vi "AMI_Measure_cDAQ.vi"(6 "error in (no error)":errorcluster, 7 "Index":i8) -> (0 "error out":errorcluster, 2 "resulting string 1":string="Set Temperatura 4.2K at 20K/min, FastSettle, Sweep&meas", 3 "Cancelled?":bool)   [LabVIEW 2017]
doc: "Use this template to create a dialog box. This template polls the state of the buttons on the front panel and does not use events. Use the Dialog Using Events template (not available in Base package) to create a dialog box with event handling."
panel:
  in  "Meas Time (s)":dbl=10.0
  in  "Measure Rate (s)":dbl=1.0 format="%.2f"
  in  "Averages":u16=10
  out "Channel 1":bool=TRUE
  out "Channel 2":bool=TRUE
  out "Channel 3":bool=TRUE
  out "Channel 4":bool=TRUE
  in  "Cancel":bool
  in  "OK":bool
  # "MEASURE cDAQ"
  # "Enero 2023 V2.1  a-sslcdms"
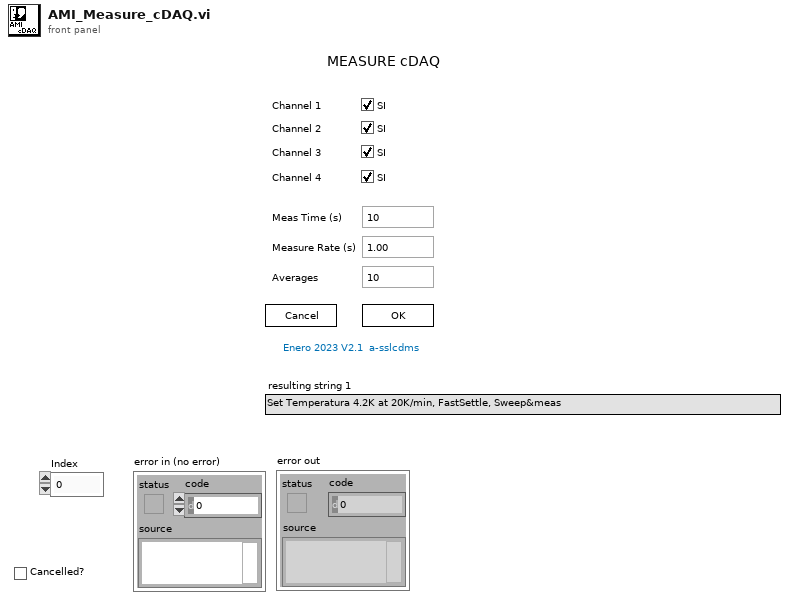
[diagram p1: front panel]
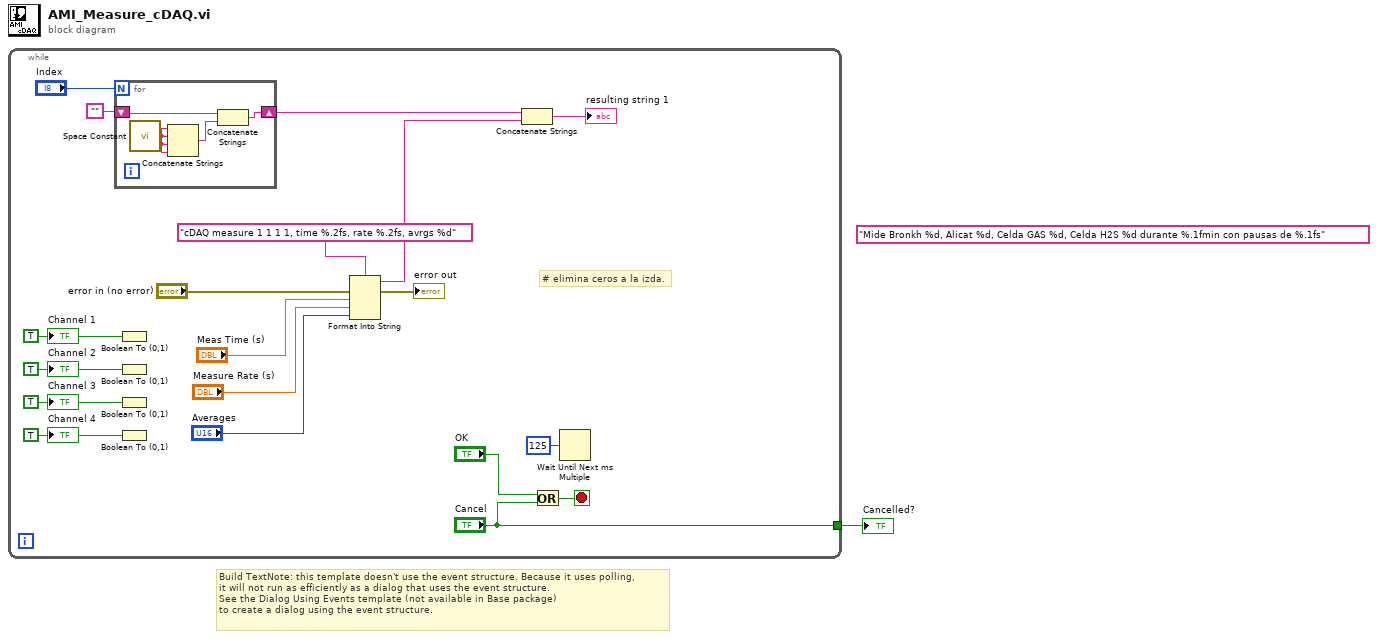
[diagram p0: block diagram]
diagram:
  (unwired) "Mide Bronkh %d, Alicat %d, Celda GAS %d, Celda H2S %d durante %.1fmin con pausas de %.1fs" ("format string")
  # "Build TextNote: this template doesn't use the event structure. Because it uses polling, \nit will not run as efficiently as a dialog that uses the event structure.\nSee the Dialog Using Events template (not available in Base package) \nto create a dialog using the event structure."
  n1 = while {
    tunnel: ["Cancel"] -> w1
    stop <- w19 stop-if-true
    w2 = TRUE ("Channel 4")
    w3 = TRUE ("Channel 3")
    w4 = TRUE ("Channel 2")
    w5 = TRUE ("Channel 1")
    # "# elimina ceros a la izda."
    n2 = for {
      N: "Index" -> [_]
      shift-right: [w23] -> w9
      shift-left: "" -> [w22]
      n3 = call <vilib>:"Space Constant.vi"() -> ("String"=w21:string)
      n4 = Concatenate Strings(w21, w21, w21, w21) -> (w24:string)
      n5 = Concatenate Strings(w22, w24) -> (w23:string)
    }
    n6 = Boolean To (0,1)(Boolean=w5) -> ()  [unwired: 1 out]
    n7 = Boolean To (0,1)(Boolean=w4) -> ()  [unwired: 1 out]
    n8 = Boolean To (0,1)(Boolean=w3) -> ()  [unwired: 1 out]
    n9 = Boolean To (0,1)(Boolean=w2) -> ()  [unwired: 1 out]
    n10 = Format Into String(format string="cDAQ measure 1 1 1 1, time %.2fs, rate %.2fs, avrgs %d", error in="error in (no error)", "Meas Time (s)", "Measure Rate (s)", "Averages") -> (resulting string=w11:string, error out=→"error out":errorcluster)  [unwired: 1 in]
    n11 = Concatenate Strings(w9, w11) -> (→"resulting string 1":string)
    n12 = Or(x="OK", y="Cancel") -> (x .or. y?=w19:bool)
    n13 = Wait Until Next ms Multiple(millisecond multiple=u32 125) -> ()  [unwired: 1 out]
    "Channel 4" <- w2
    "Channel 3" <- w3
    "Channel 1" <- w5
    "Channel 2" <- w4
  }
  "Cancelled?" <- w1
